vi "Msg Handler.vi"(11 "queue":refnum<queue>) -> (0 "error out":errorcluster)   [LabVIEW 2020, in "Multi Process.lvlib"]
uses:
  Multi Process.lvlib
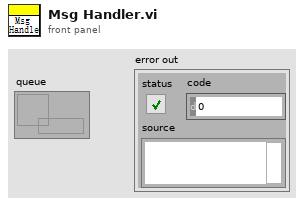
[diagram p1: front panel]
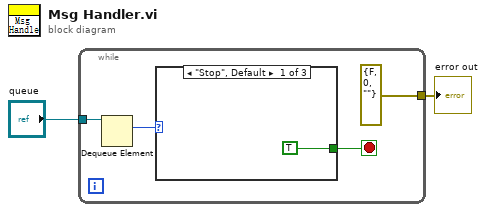
[diagram p0: block diagram]
diagram:
  n1 = while {
    tunnel: "queue" -> [w6]
    tunnel: [errorcluster {"status"=FALSE, "code"=0, "source"=""} ("error constant")] -> w1
    stop <- w4 stop-if-true
    n2 = Dequeue Element(queue=w6) -> (element=w5:enum16{"Stop", "Execute", "Initialize"})  [unwired: 2 in, 3 out]
    n3 = case shown="\"Stop\", Default" w5 {
      tunnel: [TRUE _ _] -> w4
      frame "Stop", Default {
      }
      frame "Execute" {
      }
      frame "Initialize" {
      }
    }
  }
  "error out" <- w1
